vi "TCP Connection Manager.vi"(6 "Properties In":T1, 8 "error in (no error)":errorcluster, 9 "Method":T4, 10 "Index":i32, 11 "Connection In":T2) -> (0 "error out":errorcluster, 1 "Number of Connections":i32, 2 "All Connections":T2[](array[typedef]), 3 "Connection Out":T2, 4 "Properties out":T1, 5 "All Properties":T1[](array[typedef]))   [LabVIEW 2010]
doc: "This VI maintains the list of host connections. \n\nCopyright 2015, 2016, 2017 National Instruments Corporation\n\nLicensed under the Apache License, Version 2.0 (the \"License\"); you may not use this file except in compliance with the License.\n\n You may obtain a copy of the License at\n\n http://www.apache.org/licenses/LICENSE-2.0\n\nUnless required by applicable law or agreed to in writing, software distributed under the License is distributed on an \"AS IS\" BASIS, WITHOUT WARRANTIES OR CONDITIONS OF ANY KIND, either express or implied.\n\nSee the License for the specific language governing permissions and limitations under the License."
uses:
  stm_TCPConnectionMethod.ctl
  stm_TCP Connection Info.ctl
  stm_MetaDataElement.ctl
  stm_TCPConnectionProperties.ctl
  NI STM.lvlib
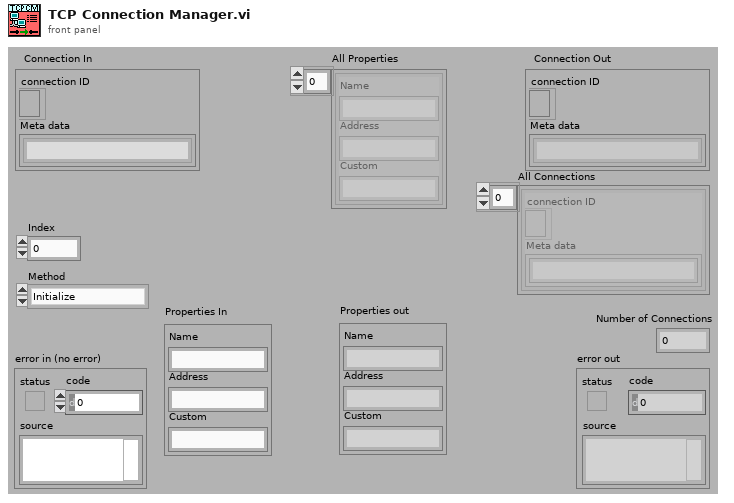
[diagram p1: front panel]
types:
  T1 = typedef "stm_TCPConnectionProperties.ctl" = cluster{"Name":string, "Address":string, "Custom":string}
  T2 = typedef "stm_TCP Connection Info.ctl" = cluster{"connection ID":refnum<k5>, "Meta data":T3[]}
  T3 = typedef "stm_MetaDataElement.ctl" = string
  T4 = typedef "stm_TCPConnectionMethod.ctl" = enum16{"Initialize", "Add Connection", "Set Properties", "Get Connection(s)", "Remove Connection", "Remove All Connections", "Get Connection Count"}
  T5 = typedef "NI STM.lvlib/TCP Connection Info.ctl" = cluster{"connection ID":refnum<k5>, "meta data":T6[]}
  T6 = typedef "NI STM.lvlib/MetaDataElement.ctl" = string
  T7 = typedef "NI STM.lvlib/TCP Connection Properties.ctl" = cluster{"Name":string, "Address":string, "Custom":string}
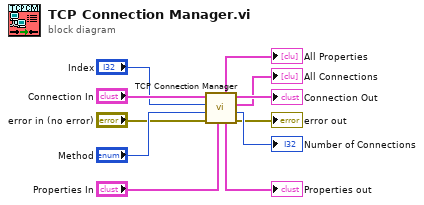
[diagram p0: block diagram]
diagram:
  n1 = call "TCP Connection Manager.vi"("properties in"="Properties In", "error in"="error in (no error)", "method"="Method", "index"="Index", "connection in"="Connection In") -> ("error out"=→"error out":errorcluster, "number of connections"=→"Number of Connections":i32, "all connections"=→"All Connections":T5[], "connection out"=→"Connection Out":T5, "properties out"=→"Properties out":T7, "all properties"=→"All Properties":T7[])  [unwired: 1 in]
